vi "CoolerONSD.vi"(2 "error in (no error)":errorcluster) -> (0 "error out":errorcluster, 1 "DLL error code":u32)   [LabVIEW 2015]
doc: "Switches ON the cooling. The rate of temperature change is controlled until the temperature is within 3 degrees of the set value. Control is returned immediately to the calling application.\n\n<B>Error codes:</B>\nDRV_SUCCESS - Temperature controller switched ON.\nDRV_NOT_INITIALIZED - System not initialized.\nDRV_ACQUIRING - Acquisition in progress.\nDRV_ERROR_ACK - Unable to communicate with card.\n\n<B>NOTES:</B>\n<B>The temperature to which the detector will be cooled is set via SetTemperature. The temperature stabilization is controlled via hardware, but the current temperature can be obtained via GetTemperature. The temperature of the sensor is gradually brought to the desired temperature to ensure no thermal stresses are set up in the sensor.</B>"
uses:
  DLL/atmcd32d.dll
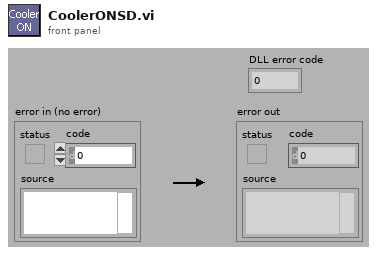
[diagram p1: front panel]
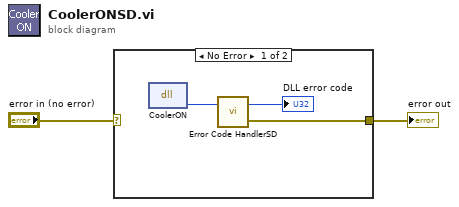
[diagram p0: block diagram]
diagram:
  n1 = case shown="No Error" "error in (no error)" {
    selector: "error in (no error)" -> [_ w6]
    tunnel: [w4 w6] -> w1
    frame No Error {
      n2 = dll-call lib="G:/SD/TRANCON-2015/DLL/Atmcd32d.dll" fn="CoolerON"() -> (w5:u32)  [unwired: 3 in, 2 out]
      n3 = call "Error Code HandlerSD.vi"("DLL error code"=w5) -> ("error out"=w4:errorcluster, "dup DLL error code"=→"DLL error code":u32)  [unwired: 1 in]
    }
    frame Error {
    }
  }
  "error out" <- w1
